vi "Upload File to Experiment (Buffer).vi"(7 "server file name":string, 8 "error in (no error)":errorcluster, 9 "file data":string, 10 "experiment id":u32, 11 "eLab in":refnum<class "PL eLabFTW Client.lvclass">) -> (0 "error out":errorcluster, 2 "file id":u32, 3 "eLab out":refnum<class "PL eLabFTW Client.lvclass">)   [LabVIEW 2015, in "PL eLabFTW Client.lvclass"]
doc: "Uploads file to the experiment and returns new file id."
uses:
  PL eLabFTW Client.lvclass
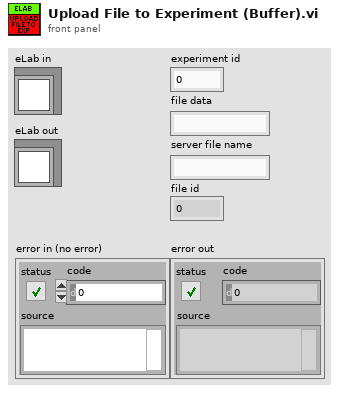
[diagram p1: front panel]
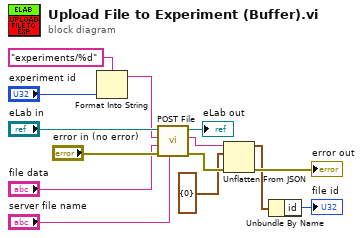
[diagram p0: block diagram]
diagram:
  n1 = Format Into String(format string="experiments/%d", "experiment id") -> (resulting string=w9:string)  [unwired: 2 in, 1 out]
  n2 = call "POST File.vi"("server file name"="server file name", "error in (no error)"="error in (no error)", "buffer"="file data", "relative URL"=w9, "eLab in"="eLab in") -> ("error out"=w5:errorcluster, "response body"=w4:string, "eLab out"=→"eLab out":refnum<class "PL eLabFTW Client.lvclass">)  [unwired: 4 in]
  n3 = Unflatten From JSON(JSON string=w4, type and defaults=cluster{"id":u32} {"id"=0}, error in (no error)=w5) -> (value=w1:cluster{"id":u32}, error out=→"error out":errorcluster)  [unwired: 4 in]
  n4 = Unbundle By Name(w1) -> ("id"=→"file id":u32)
